vi "Transmit User Info.vi"(3 "错误输入":errorcluster, 4 "Password":refnum<vi>, 5 "UserName":refnum<vi>) -> (0 "error out":errorcluster)   [LabVIEW 2013]
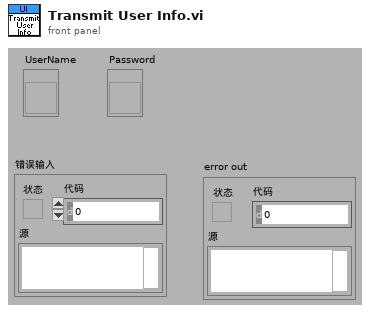
[diagram p1: front panel]
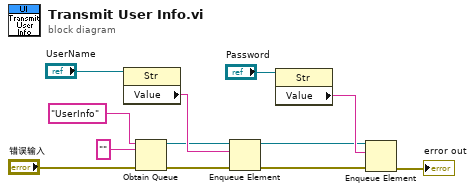
[diagram p0: block diagram]
diagram:
  n1 = property class="Str"(reference="UserName") -> ("Value"=w8:string)  [unwired: 1 in, 2 out]
  n2 = Obtain Queue(name (unnamed)="UserInfo" ("名称（未命名）"), element data type="" ("名称（未命名）"), error in (no error)="错误输入") -> (queue out=w5:refnum<queue>, error out=w6:errorcluster)  [unwired: 2 in, 1 out]
  n3 = Enqueue Element(queue=w5, element=w8, error in (no error)=w6) -> (queue out=w9:refnum<queue>, error out=w10:errorcluster)  [unwired: 1 in, 1 out]
  n4 = property class="Str"(reference="Password") -> ("Value"=w11:string)  [unwired: 1 in, 2 out]
  n5 = Enqueue Element(queue=w9, element=w11, error in (no error)=w10) -> (error out=→"error out":errorcluster)  [unwired: 1 in, 2 out]
